vi "refresh group data.vi"(8 "error in":errorcluster, 9 "specification":T1[](array[typedef]), 10 "group in":T3, 11 "data table in":T3) -> (0 "error out":errorcluster, 2 "group out":T3, 3 "data table out":T3)   [LabVIEW 2013, in "tag bus.lvlib" / "data table.lvlib"]
doc: "Accepts a primary data table and a subgroup data table, and copies data from the main table into the group."
uses:
  data table.lvlib
  data table.ctl
  group specification.ctl
  tag/Data Type.ctl
  data polymorphs/read many/read Doubles.vi
  data polymorphs/write all/write all Doubles.vi
  data polymorphs/read many/read I64s.vi
  data polymorphs/write all/write all I64s.vi
  data polymorphs/read many/read Singles.vi
  data polymorphs/write all/write all Singles.vi
  data polymorphs/read many/read I8s.vi
  data polymorphs/write all/write all I8s.vi
  data polymorphs/read many/read U64s.vi
  data polymorphs/write all/write all U64s.vi
  data polymorphs/read many/read U32s.vi
  data polymorphs/write all/write all U32s.vi
  data polymorphs/read many/read U16s.vi
  data polymorphs/write all/write all U16s.vi
  data polymorphs/read many/read U8s.vi
  data polymorphs/write all/write all U8s.vi
  data polymorphs/read many/read Strings.vi
  data polymorphs/write all/write all Strings.vi
  data polymorphs/read many/read Booleans.vi
  data polymorphs/write all/write all Booleans.vi
  data polymorphs/read many/read Array of U8s.vi
  data polymorphs/write all/write all Array of U8s.vi
  data polymorphs/read many/read Array of U16s.vi
  data polymorphs/write all/write all Array of U16s.vi
  data polymorphs/read many/read Array of U32s.vi
  data polymorphs/write all/write all Array of U32s.vi
  data polymorphs/read many/read Array of U64s.vi
  data polymorphs/write all/write all Array of U64s.vi
  data polymorphs/read many/read Array of I64s.vi
  data polymorphs/write all/write all Array of I64s.vi
  data polymorphs/read many/read Array of I32s.vi
  data polymorphs/write all/write all Array of I32s.vi
  data polymorphs/read many/read Array of I16s.vi
  data polymorphs/write all/write all Array of I16s.vi
  data polymorphs/read many/read Array of I8s.vi
  data polymorphs/write all/write all Array of I8s.vi
  data polymorphs/read many/read Array of Doubles.vi
  data polymorphs/write all/write all Array of Doubles.vi
  data polymorphs/read many/read Array of Singles.vi
  data polymorphs/write all/write all Array of Singles.vi
  data polymorphs/read many/read Array of Booleans.vi
  data polymorphs/write all/write all Array of Booleans.vi
  data polymorphs/read many/read Array of Strings.vi
  data polymorphs/write all/write all Array of Strings.vi
  tag bus error generator.vi
  tag/tag descriptor.lvclass
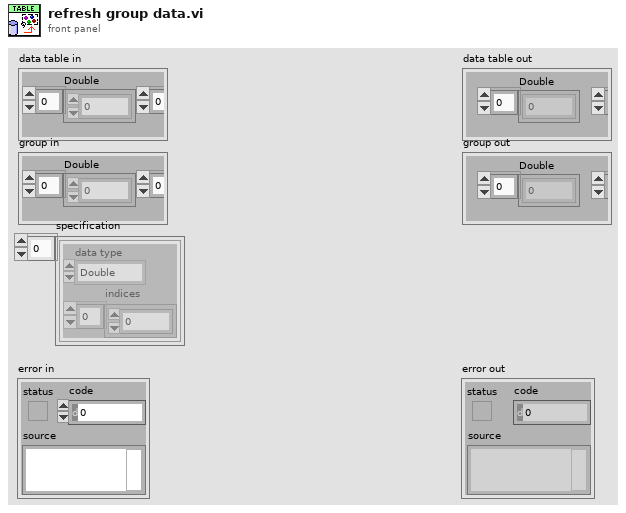
[diagram p1: front panel]
types:
  T1 = typedef "tag bus.lvlib/data table.lvlib/group specification.ctl" = cluster{"data type":T2, "indices":i32[]}
  T2 = typedef "tag bus.lvlib/tag descriptor.lvclass/Data Type.ctl" = enum16{"Double", "Single", "I64", "I32", "I16", "I8", "U64", "U32", "U16", "U8", "Boolean", "String", "Array of Double", "Array of Single", "Array of I64", "Array of I32", "Array of I16", "Array of I8", "Array of U64", "Array of U32", "Array of U16", "Array of U8", "Array of Boolean", "Array of String"}
  T3 = typedef "tag bus.lvlib/data table.lvlib/data table.ctl" = cluster{"Double":dbl[], "Single":sgl[], "I64":i64[], "I32":i32[], "I16":i16[], "I8":i8[], "U64":u64[], "U32":u32[], "U16":u16[], "U8":u8[], "Boolean":bool[], "String":string[], "Array of Double":cluster{"DBL Array":dbl[]}[], "Array of Single":cluster{"SGL Array":sgl[]}[], "Array of I64":cluster{"I64 Array":i64[]}[], "Array of I32":cluster{"I32 Array":i32[]}[], "Array of I16":cluster{"I16 Array":i16[]}[], "Array of I8":cluster{"I8 Array":i8[]}[], "Array of U64":cluster{"U64 Array":u64[]}[], "Array of U32":cluster{"U32 Array":u32[]}[], "Array of U16":cluster{"U16 Array":u16[]}[], "Array of U8":cluster{"U8 Array":u8[]}[], "Array of Boolean":cluster{"Boolean Array":bool[]}[], "Array of String":cluster{"String Array":string[]}[]}
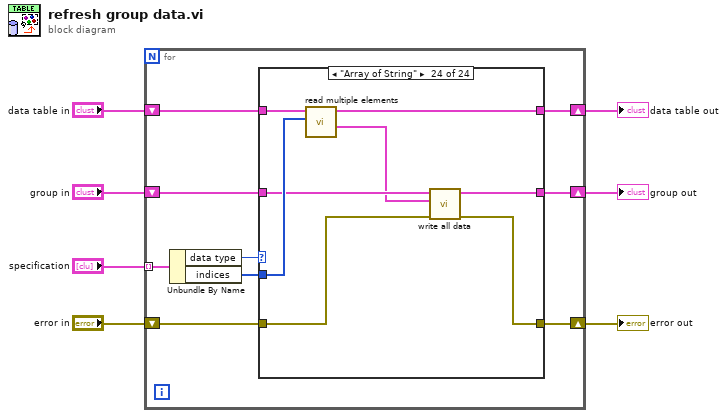
[diagram p0: block diagram]
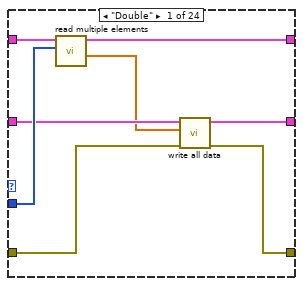
[diagram p2: hidden frame]
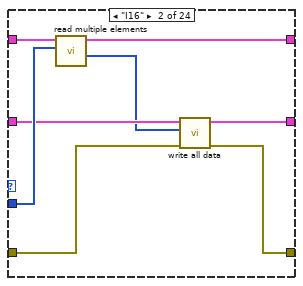
[diagram p3: hidden frame]
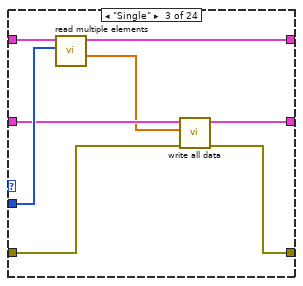
[diagram p4: hidden frame]
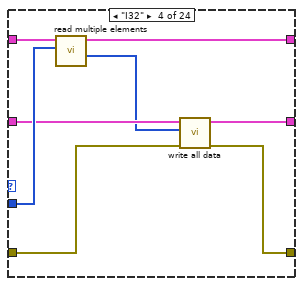
[diagram p5: hidden frame]
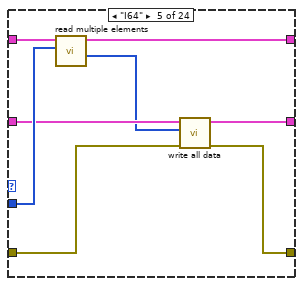
[diagram p6: hidden frame]
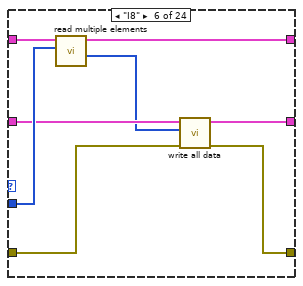
[diagram p7: hidden frame]
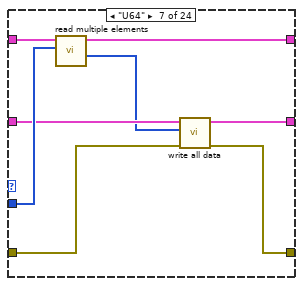
[diagram p8: hidden frame]
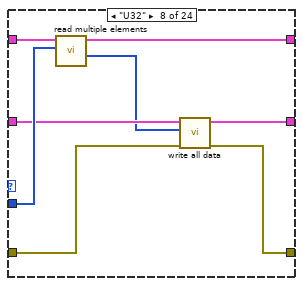
[diagram p9: hidden frame]
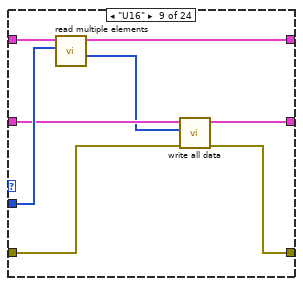
[diagram p10: hidden frame]
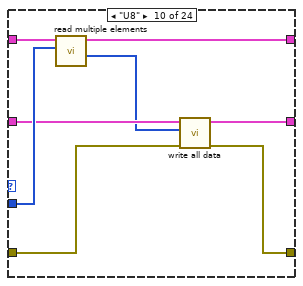
[diagram p11: hidden frame]
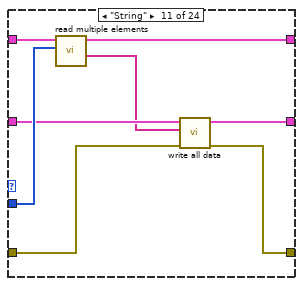
[diagram p12: hidden frame]
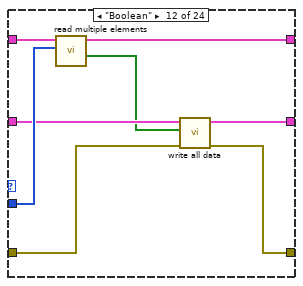
[diagram p13: hidden frame]
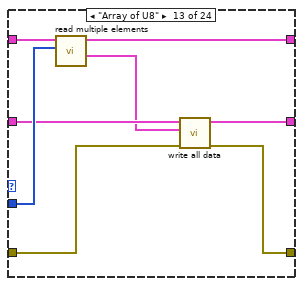
[diagram p14: hidden frame]
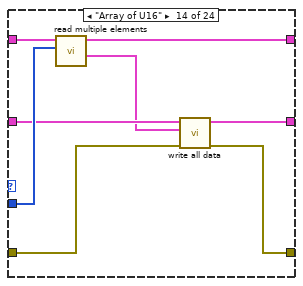
[diagram p15: hidden frame]
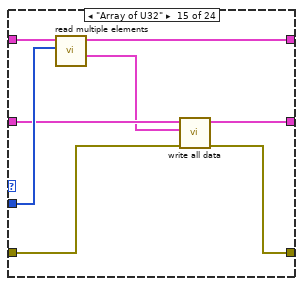
[diagram p16: hidden frame]
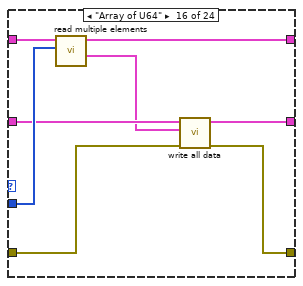
[diagram p17: hidden frame]
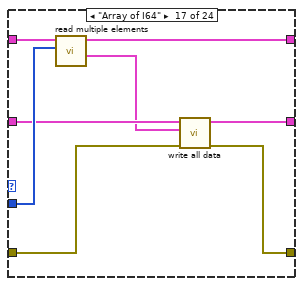
[diagram p18: hidden frame]
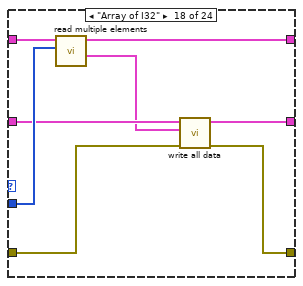
[diagram p19: hidden frame]
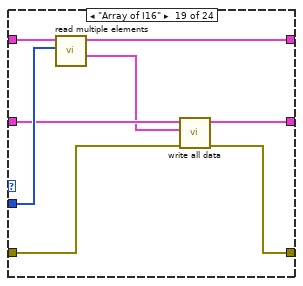
[diagram p20: hidden frame]
diagram:
  n1 = for {
    shift-right: [w11] -> w4
    shift-left: "error in" -> [w10]
    shift-right: [w12] -> w5
    shift-left: "data table in" -> [w13]
    shift-right: [w8] -> w2
    shift-left: "group in" -> [w9]
    tunnel: "specification" -> [w16] mode=indexing
    n2 = Unbundle By Name(w16) -> ("data type"=w15:T2, "indices"=w14:i32[])
    n3 = case shown="\"Array of String\"" w15 {
      tunnel: w14 -> [w22 w30 w38 w46 w54 w62 w70 w78 w86 w94 w102 w110 w118 w126 w134 w142 w150 w158 w166 w174 w182 w190 w198 w206]
      tunnel: w13 -> [w24 w32 w40 w48 w56 w64 w72 w80 w88 w96 w104 w112 w120 w128 w136 w144 w152 w160 w168 w176 w184 w192 w200 w208]
      tunnel: [w23 w31 w39 w47 w55 w63 w71 w79 w87 w95 w103 w111 w119 w127 w135 w143 w151 w159 w167 w175 w183 w191 w199 w207] -> w12
      tunnel: [w19 w27 w35 w43 w51 w59 w67 w75 w83 w91 w99 w107 w115 w123 w131 w139 w147 w155 w163 w171 w179 w187 w195 w203] -> w11
      tunnel: w10 -> [w20 w28 w36 w44 w52 w60 w68 w76 w84 w92 w100 w108 w116 w124 w132 w140 w148 w156 w164 w172 w180 w188 w196 w204]
      tunnel: w9 -> [w21 w29 w37 w45 w53 w61 w69 w77 w85 w93 w101 w109 w117 w125 w133 w141 w149 w157 w165 w173 w181 w189 w197 w205]
      tunnel: [w18 w26 w34 w42 w50 w58 w66 w74 w82 w90 w98 w106 w114 w122 w130 w138 w146 w154 w162 w170 w178 w186 w194 w202] -> w8
      frame "Double" {
        n4 = call-poly "read multiple elements.vi"("indices"=w22, "data table in"=w24) -> ("values"=w17:dbl[], "data table out"=w23:T3)  [unwired: 8 in]
        n5 = call-poly "write all data.vi"("error in"=w20, "values"=w17, "data table in"=w21) -> ("error out"=w19:errorcluster, "data table out"=w18:T3)  [unwired: 7 in]
      }
      frame "I16" {
        n6 = call-poly "read multiple elements.vi"("indices"=w30, "data table in"=w32) -> ("values"=w25:i64[], "data table out"=w31:T3)  [unwired: 8 in]
        n7 = call-poly "write all data.vi"("error in"=w28, "values"=w25, "data table in"=w29) -> ("error out"=w27:errorcluster, "data table out"=w26:T3)  [unwired: 7 in]
      }
      frame "Single" {
        n8 = call-poly "read multiple elements.vi"("indices"=w38, "data table in"=w40) -> ("values"=w33:sgl[], "data table out"=w39:T3)  [unwired: 8 in]
        n9 = call-poly "write all data.vi"("error in"=w36, "values"=w33, "data table in"=w37) -> ("error out"=w35:errorcluster, "data table out"=w34:T3)  [unwired: 7 in]
      }
      frame "I32" {
        n10 = call-poly "read multiple elements.vi"("indices"=w46, "data table in"=w48) -> ("values"=w41:i64[], "data table out"=w47:T3)  [unwired: 8 in]
        n11 = call-poly "write all data.vi"("error in"=w44, "values"=w41, "data table in"=w45) -> ("error out"=w43:errorcluster, "data table out"=w42:T3)  [unwired: 7 in]
      }
      frame "I64" {
        n12 = call-poly "read multiple elements.vi"("indices"=w54, "data table in"=w56) -> ("values"=w49:i64[], "data table out"=w55:T3)  [unwired: 8 in]
        n13 = call-poly "write all data.vi"("error in"=w52, "values"=w49, "data table in"=w53) -> ("error out"=w51:errorcluster, "data table out"=w50:T3)  [unwired: 7 in]
      }
      frame "I8" {
        n14 = call-poly "read multiple elements.vi"("indices"=w62, "data table in"=w64) -> ("values"=w57:i8[], "data table out"=w63:T3)  [unwired: 8 in]
        n15 = call-poly "write all data.vi"("error in"=w60, "values"=w57, "data table in"=w61) -> ("error out"=w59:errorcluster, "data table out"=w58:T3)  [unwired: 7 in]
      }
      frame "U64" {
        n16 = call-poly "read multiple elements.vi"("indices"=w70, "data table in"=w72) -> ("values"=w65:u64[], "data table out"=w71:T3)  [unwired: 8 in]
        n17 = call-poly "write all data.vi"("error in"=w68, "values"=w65, "data table in"=w69) -> ("error out"=w67:errorcluster, "data table out"=w66:T3)  [unwired: 7 in]
      }
      frame "U32" {
        n18 = call-poly "read multiple elements.vi"("indices"=w78, "data table in"=w80) -> ("values"=w73:u32[], "data table out"=w79:T3)  [unwired: 8 in]
        n19 = call-poly "write all data.vi"("error in"=w76, "values"=w73, "data table in"=w77) -> ("error out"=w75:errorcluster, "data table out"=w74:T3)  [unwired: 7 in]
      }
      frame "U16" {
        n20 = call-poly "read multiple elements.vi"("indices"=w86, "data table in"=w88) -> ("values"=w81:u16[], "data table out"=w87:T3)  [unwired: 8 in]
        n21 = call-poly "write all data.vi"("error in"=w84, "values"=w81, "data table in"=w85) -> ("error out"=w83:errorcluster, "data table out"=w82:T3)  [unwired: 7 in]
      }
      frame "U8" {
        n22 = call-poly "read multiple elements.vi"("indices"=w94, "data table in"=w96) -> ("values"=w89:u8[], "data table out"=w95:T3)  [unwired: 8 in]
        n23 = call-poly "write all data.vi"("error in"=w92, "values"=w89, "data table in"=w93) -> ("error out"=w91:errorcluster, "data table out"=w90:T3)  [unwired: 7 in]
      }
      frame "String" {
        n24 = call-poly "read multiple elements.vi"("indices"=w102, "data table in"=w104) -> ("values"=w97:string[], "data table out"=w103:T3)  [unwired: 8 in]
        n25 = call-poly "write all data.vi"("error in"=w100, "values"=w97, "data table in"=w101) -> ("error out"=w99:errorcluster, "data table out"=w98:T3)  [unwired: 7 in]
      }
      frame "Boolean" {
        n26 = call-poly "read multiple elements.vi"("indices"=w110, "data table in"=w112) -> ("values"=w105:bool[], "data table out"=w111:T3)  [unwired: 8 in]
        n27 = call-poly "write all data.vi"("error in"=w108, "values"=w105, "data table in"=w109) -> ("error out"=w107:errorcluster, "data table out"=w106:T3)  [unwired: 7 in]
      }
      frame "Array of U8" {
        n28 = call-poly "read multiple elements.vi"("indices"=w118, "data table in"=w120) -> ("values"=w113:cluster{"Array":u8[]}[], "data table out"=w119:T3)  [unwired: 8 in]
        n29 = call-poly "write all data.vi"("error in"=w116, "values"=w113, "data table in"=w117) -> ("error out"=w115:errorcluster, "data table out"=w114:T3)  [unwired: 7 in]
      }
      frame "Array of U16" {
        n30 = call-poly "read multiple elements.vi"("indices"=w126, "data table in"=w128) -> ("values"=w121:cluster{"Array":u16[]}[], "data table out"=w127:T3)  [unwired: 8 in]
        n31 = call-poly "write all data.vi"("error in"=w124, "values"=w121, "data table in"=w125) -> ("error out"=w123:errorcluster, "data table out"=w122:T3)  [unwired: 7 in]
      }
      frame "Array of U32" {
        n32 = call-poly "read multiple elements.vi"("indices"=w134, "data table in"=w136) -> ("values"=w129:cluster{"Array":u32[]}[], "data table out"=w135:T3)  [unwired: 8 in]
        n33 = call-poly "write all data.vi"("error in"=w132, "values"=w129, "data table in"=w133) -> ("error out"=w131:errorcluster, "data table out"=w130:T3)  [unwired: 7 in]
      }
      frame "Array of U64" {
        n34 = call-poly "read multiple elements.vi"("indices"=w142, "data table in"=w144) -> ("values"=w137:cluster{"Array":u64[]}[], "data table out"=w143:T3)  [unwired: 8 in]
        n35 = call-poly "write all data.vi"("error in"=w140, "values"=w137, "data table in"=w141) -> ("error out"=w139:errorcluster, "data table out"=w138:T3)  [unwired: 7 in]
      }
      frame "Array of I64" {
        n36 = call-poly "read multiple elements.vi"("indices"=w150, "data table in"=w152) -> ("values"=w145:cluster{"Array":i64[]}[], "data table out"=w151:T3)  [unwired: 8 in]
        n37 = call-poly "write all data.vi"("error in"=w148, "values"=w145, "data table in"=w149) -> ("error out"=w147:errorcluster, "data table out"=w146:T3)  [unwired: 7 in]
      }
      frame "Array of I32" {
        n38 = call-poly "read multiple elements.vi"("indices"=w158, "data table in"=w160) -> ("values"=w153:cluster{"Array":i32[]}[], "data table out"=w159:T3)  [unwired: 8 in]
        n39 = call-poly "write all data.vi"("error in"=w156, "values"=w153, "data table in"=w157) -> ("error out"=w155:errorcluster, "data table out"=w154:T3)  [unwired: 7 in]
      }
      frame "Array of I16" {
        n40 = call-poly "read multiple elements.vi"("indices"=w166, "data table in"=w168) -> ("values"=w161:cluster{"Array":i16[]}[], "data table out"=w167:T3)  [unwired: 8 in]
        n41 = call-poly "write all data.vi"("error in"=w164, "values"=w161, "data table in"=w165) -> ("error out"=w163:errorcluster, "data table out"=w162:T3)  [unwired: 7 in]
      }
      frame "Array of I8" {
        n42 = call-poly "read multiple elements.vi"("indices"=w174, "data table in"=w176) -> ("values"=w169:cluster{"Array":i8[]}[], "data table out"=w175:T3)  [unwired: 8 in]
        n43 = call-poly "write all data.vi"("error in"=w172, "values"=w169, "data table in"=w173) -> ("error out"=w171:errorcluster, "data table out"=w170:T3)  [unwired: 7 in]
      }
      frame "Array of Double" {
        n44 = call-poly "read multiple elements.vi"("indices"=w182, "data table in"=w184) -> ("values"=w177:cluster{"Array":dbl[]}[], "data table out"=w183:T3)  [unwired: 8 in]
        n45 = call-poly "write all data.vi"("error in"=w180, "values"=w177, "data table in"=w181) -> ("error out"=w179:errorcluster, "data table out"=w178:T3)  [unwired: 7 in]
      }
      frame "Array of Single" {
        n46 = call-poly "read multiple elements.vi"("indices"=w190, "data table in"=w192) -> ("values"=w185:cluster{"Array":sgl[]}[], "data table out"=w191:T3)  [unwired: 8 in]
        n47 = call-poly "write all data.vi"("error in"=w188, "values"=w185, "data table in"=w189) -> ("error out"=w187:errorcluster, "data table out"=w186:T3)  [unwired: 7 in]
      }
      frame "Array of Boolean" {
        n48 = call-poly "read multiple elements.vi"("indices"=w198, "data table in"=w200) -> ("values"=w193:cluster{"Array":bool[]}[], "data table out"=w199:T3)  [unwired: 8 in]
        n49 = call-poly "write all data.vi"("error in"=w196, "values"=w193, "data table in"=w197) -> ("error out"=w195:errorcluster, "data table out"=w194:T3)  [unwired: 7 in]
      }
      frame "Array of String" {
        n50 = call-poly "read multiple elements.vi"("indices"=w206, "data table in"=w208) -> ("values"=w201:cluster{"Array":string[]}[], "data table out"=w207:T3)  [unwired: 8 in]
        n51 = call-poly "write all data.vi"("error in"=w204, "values"=w201, "data table in"=w205) -> ("error out"=w203:errorcluster, "data table out"=w202:T3)  [unwired: 7 in]
      }
    }
  }
  "error out" <- w4
  "data table out" <- w5
  "group out" <- w2
